vi "Read Transfer Groups.vi"(8 "error in (no error)":errorcluster, 11 "Plugin Configuration in":refnum<class "Plugin Configuration.lvclass">) -> (0 "error out":errorcluster, 2 "Transfer Groups":refnum<class "Configuration.Transfer Group.lvclass">[](array[class]), 3 "Plugin Configuration out":refnum<class "Plugin Configuration.lvclass">)   [LabVIEW 2016, in "Plugin Configuration.lvclass"]
uses:
  Plugin Configuration.lvclass
  Configuration.Transfer Group/Configuration.Transfer Group.lvclass
  Plugin Configuration.lvclass/Plugin Configuration.ctl
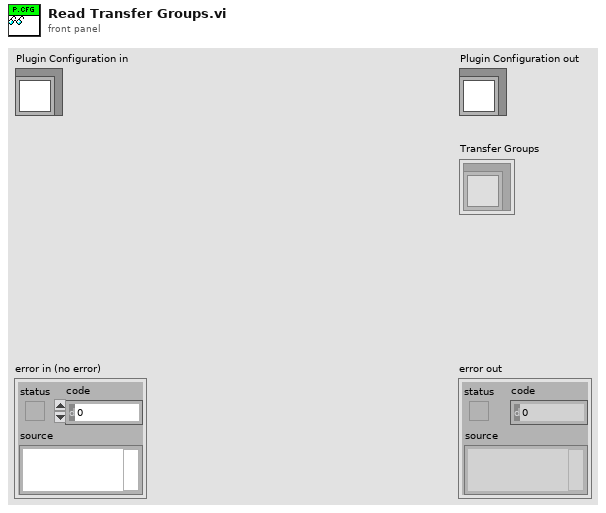
[diagram p1: front panel]
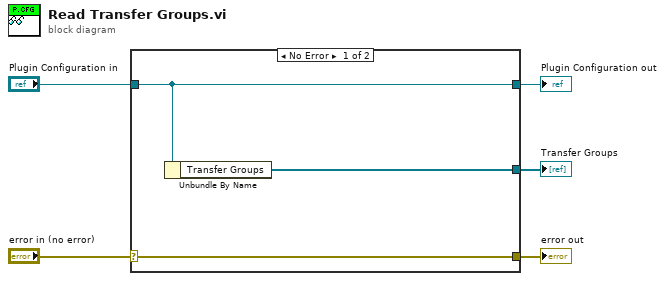
[diagram p0: block diagram]
diagram:
  n1 = case shown="No Error" "error in (no error)" {
    selector: "error in (no error)" -> [w8 w9]
    tunnel: [w8 w9] -> w4
    tunnel: [w7 w10] -> w2
    tunnel: "Plugin Configuration in" -> [w7 w10]
    tunnel: [w6 _] -> w1
    frame No Error {
      n2 = Unbundle By Name(w7) -> ("Transfer Groups"=w6:refnum<class "Configuration.Transfer Group.lvclass">[])
    }
    frame Error {
    }
  }
  "error out" <- w4
  "Plugin Configuration out" <- w2
  "Transfer Groups" <- w1
